vi "serial_arduino_ABC.vi"() -> ()   [LabVIEW 2015]
uses:
  <vilib>/Instr/_visa.llb/VISA Configure Serial Port (Instr).vi
panel:
  out "Voltage":dbl
  out "Waveform Chart":dbl(graph)
  in  "flow control":u16(ring) items=["None"=0, "XON/XOFF"=1, "RTS/CTS"=2, "DTR/DSR"=4]
  in  "stop bits":u16(ring)=10 items=["1.0"=10, "1.5"=15, "2.0"=20]
  in  "parity":u16(ring) items=["None", "Odd", "Even", "Mark", "Space"]
  in  "data bits":u16=8 min=5 max=8 step=1
  in  "VISA resource name":refnum<visa-resource-name>="COM1"
  in  "baud rate":u32=9600
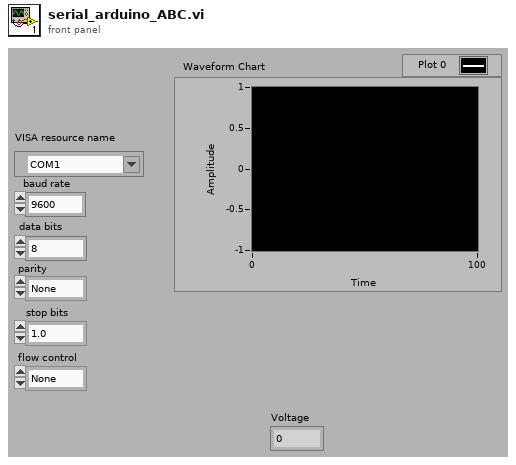
[diagram p1: front panel]
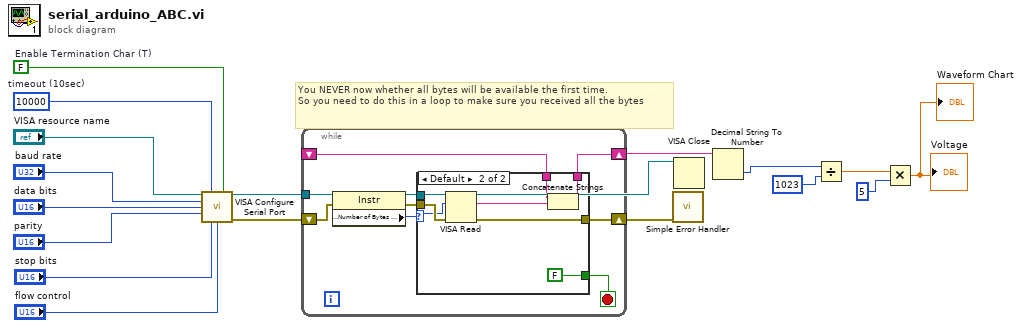
[diagram p0: block diagram]
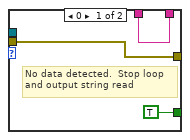
[diagram p2: hidden frame]
diagram:
  w13 = FALSE  # Enable Termination Char (T)
  w14 = u32 10000  # timeout (10sec)
  # "You NEVER now whether all bytes will be available the first time.\nSo you need to do this in a loop to make sure you received all the bytes"
  n1 = call-poly "VISA Configure Serial Port"("VISA resource name"="VISA resource name", "timeout (10sec)"=w14, "Enable Termination\nChar (T)"=w13, "baud rate (9600)"="baud rate", "data bits (8)"="data bits", "parity (0:none)"="parity", "stop bits (10: 1 bit)"="stop bits", "flow control (0:none)"="flow control") -> ("VISA resource name out"=w1:refnum<visa-resource-name>, "error out"=w4:errorcluster)  [unwired: 1 in, 5 out]
  n2 = while {
    tunnel: w1 -> [w26]
    shift-right: [w22] -> w2
    shift-left: _ -> [w23]
    shift-right: [w19] -> w3
    shift-left: w4 -> [w18]
    stop <- w24 stop-if-true
    n3 = property class="Instr"(reference=w26, error in=w18) -> (reference out=w21:refnum<visa-resource-name>, error out=w20:errorcluster, "Serial Settings:Number of Bytes at Serial Port"=w25:u32)
    n4 = case shown="Default" w25 {
      selector: w25 -> [_ w31]
      tunnel: [TRUE FALSE] -> w24
      tunnel: w23 -> [w28 w35]
      tunnel: [w28 w36] -> w22
      tunnel: w21 -> [_ w37]
      tunnel: w20 -> [w27 w32]
      tunnel: [w27 w30] -> w19
      frame 0 {
        # "No data detected.  Stop loop\nand output string read"
      }
      frame Default {
        n5 = VISA Read(VISA resource name=w37, byte count=w31, error in (no error)=w32) -> (read buffer=w34:string, error out=w30:errorcluster)  [unwired: 2 out]
        n6 = Concatenate Strings(w35, w34) -> (w36:string)
      }
    }
  }
  n7 = call <vilib>:"Simple Error Handler.vi"("error in (no error)"=w3) -> ()  [unwired: 1 in, 8 out]
  n8 = VISA Close(VISA resource name=w1) -> ()  [unwired: 1 in, 1 out]
  n9 = Decimal String To Number(string=w2) -> (number=w9:i32)  [unwired: 1 in, 2 out]
  n10 = Divide(x=w9, y=1023) -> (x/y=w7:dbl)
  n11 = Multiply(x=w7, y=5) -> (x*y=→"Waveform Chart" →"Voltage":dbl)
